vi "Keithley2400series_s2.vi"() -> ()   [LabVIEW 2010]
uses:
  <vilib>/Utility/file.llb/Write To Spreadsheet File (string).vi
  Софт/Keithley 24XX/Keithley 24XX.lvlib
panel:
  out "SEEcount":dbl
  in  "ОРЭ_th":dbl format="%.2f"
  out "Замер":dbl
  in  "stop":bool
  in  "Source Mode  (0: Voltage)":u16(ring) items=["Voltage", "Current"]
  in  "VISA resource name 2":refnum<visa-resource-name>
  in  "Serial Configuration":T1={"Baud Rate"=9600, "Parity"=0, "Data Bits"=8, "Stop Bits"=10, "Flow Control"=0} {"Flow Control" items=["None", "XON/XOFF", "RTS/CTS", "XON/XOFF & RTS/CTS", "DTR/DSR", "XON/XOFF & DTR/DSR"]; "Stop Bits" items=["1.0"=10, "1.5"=15, "2.0"=20]; "Data Bits" items=["7"=7, "8"=8]; "Parity" items=["None", "Odd", "Even", "Mark", "Space"]; "Baud Rate" items=["300"=300, "600"=600, "1200"=1200, "2400"=2400, "4800"=4800, "9600"=9600, "19200"=19200]}
  in  "Файл записи замеров":path
  in  "Ограничение":dbl format="%.2f"
  in  "Выход":dbl
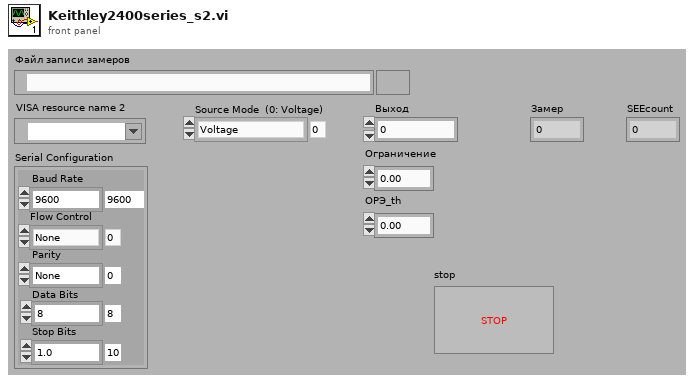
[diagram p1: front panel]
types:
  T1 = cluster{"Baud Rate":u32, "Parity":u16, "Data Bits":u16, "Stop Bits":u16, "Flow Control":u16}
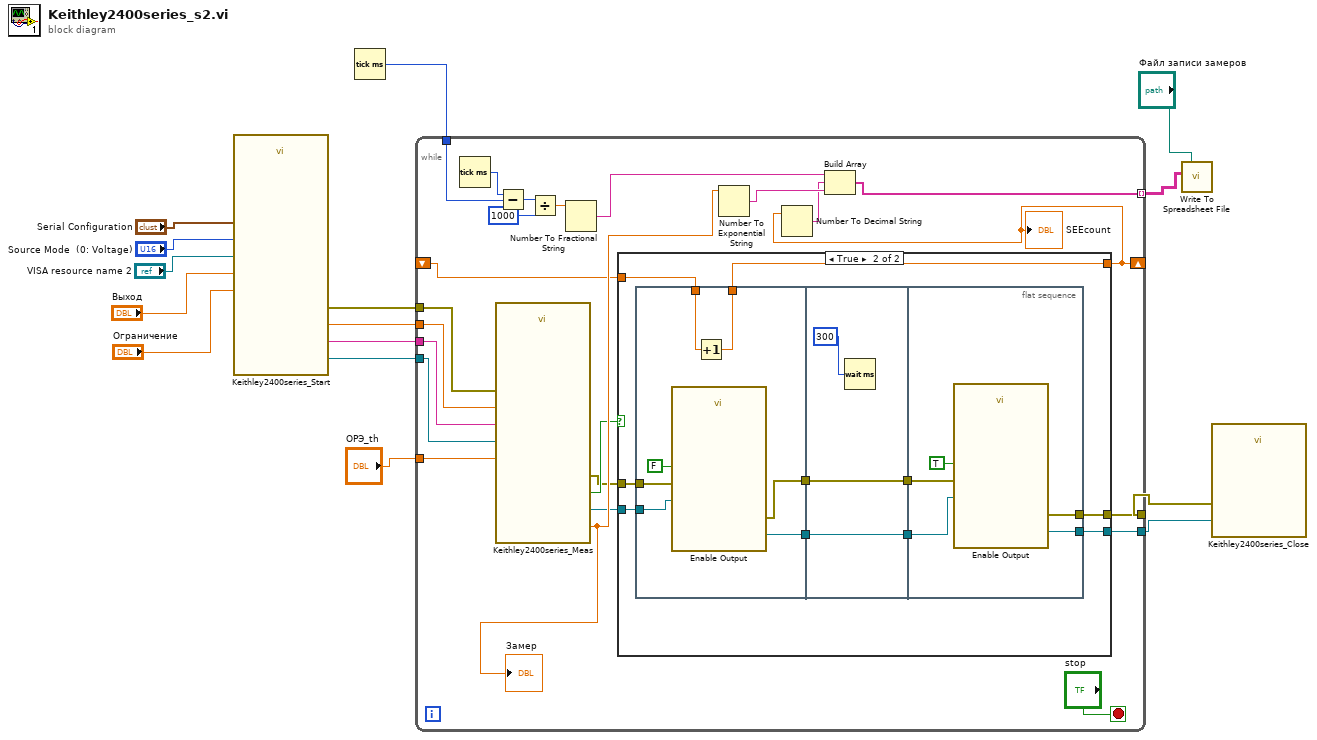
[diagram p0: block diagram]
diagram:
  n1 = call "Keithley2400series_Start.vi"("Serial Configuration"="Serial Configuration", "Source Mode  (0: Voltage) 2"="Source Mode  (0: Voltage)", "Ограничение"="Ограничение", "Выход"="Выход", "VISA resource name"="VISA resource name 2") -> ("error out"=w9:errorcluster, "MEAS:Out"=w7:string, "MEAS mode 0,Volt"=w8:dbl, "VISA resource name out"=w6:refnum<visa-resource-name>)
  n2 = Tick Count (ms)() -> (millisecond timer value=w10:u32)
  n3 = while {
    tunnel: w10 -> [w34]
    tunnel: w9 -> [w21]
    tunnel: w8 -> [w22]
    tunnel: w7 -> [w23]
    tunnel: w6 -> [w24]
    tunnel: [w19] -> w5 mode=indexing
    tunnel: "ОРЭ_th" -> [w30]
    tunnel: [w26] -> w3
    tunnel: [w25] -> w2
    shift-right: [w17] -> _
    shift-left: _ -> [w18]
    stop <- "stop" stop-if-true
    n4 = Tick Count (ms)() -> (millisecond timer value=w38:u32)
    n5 = call "Keithley2400series_Meas.vi"("MEAS:<f>"=w23, "error in (no error)"=w21, "MEAS mode, 0 Volt"=w22, "ОРЭ_th"=w30, "VISA resource name in"=w24) -> ("error out"=w27:errorcluster, "SEE"=w29:bool, "Замер"=w31:dbl, "VISA out"=w28:refnum<visa-resource-name>)
    "Замер" <- w31
    n6 = Subtract(x=w38, y=w34) -> (x-y=w37:u32)
    n7 = Divide(x=w37, y=u32 1000) -> (x/y=w35:dbl)
    n8 = Number To Fractional String(number=w35) -> (F-format string=w33:string)  [unwired: 3 in]
    n9 = case shown="True" w29 {
      tunnel: w28 -> [w41 w51]
      tunnel: w27 -> [w40 w50]
      tunnel: [w40 w45] -> w26
      tunnel: [w41 w44] -> w25
      tunnel: [w39 w43] -> w17
      tunnel: w18 -> [w39 w42]
      frame False {
      }
      frame True {
        n10 = flat-sequence {
          tunnel: w51 -> [w57]
          tunnel: w50 -> [w56]
          tunnel: [w55] -> w48
          tunnel: [w54] -> w46
          tunnel: [w53] -> w43
          tunnel: w42 -> [w52]
          tunnel: [w60] -> w49
          tunnel: w48 -> [w60]
          tunnel: [w59] -> w47
          tunnel: w46 -> [w59]
          tunnel: w49 -> [w65]
          tunnel: w47 -> [w64]
          tunnel: [w63] -> w45
          tunnel: [w62] -> w44
          frame #0 {
            n11 = call "Enable Output.vi"("error in (no error)"=w56, "Enable Output (T: Enable)"=FALSE, "VISA resource name"=w57) -> ("error out"=w55:errorcluster, "VISA resource name out"=w54:refnum<visa-resource-name>)  [unwired: 7 in]
            n12 = Increment(x=w52) -> (x+1=w53:dbl)
          }
          frame #1 {
            n13 = Wait (ms)(milliseconds to wait=u32 300) -> ()  [unwired: 1 out]
          }
          frame #2 {
            n14 = call "Enable Output.vi"("error in (no error)"=w65, "Enable Output (T: Enable)"=TRUE, "VISA resource name"=w64) -> ("error out"=w63:errorcluster, "VISA resource name out"=w62:refnum<visa-resource-name>)  [unwired: 7 in]
          }
        }
      }
    }
    "SEEcount" <- w17
    n15 = Number To Exponential String(number=w31) -> (E-format string=w20:string)  [unwired: 3 in]
    n16 = Number To Decimal String(number=w17) -> (decimal integer string=w16:string)  [unwired: 1 in]
    n17 = Build Array(w33, w16, w20) -> (w19:string[])
  }
  n18 = call-poly <vilib>:"Write To Spreadsheet File.vi"("2D data"=w5, "file path (dialog if empty)"="Файл записи замеров") -> ()  [unwired: 6 in, 1 out]
  n19 = call "Keithley2400series_Close.vi"("error in (no error)"=w3, "VISA resource name"=w2) -> ()
